vi "pessimize_adjust_bias.vi"(10 "X at maximum":dbl[](array[numeric]), 11 "Pessimize fun info":T1 {"Point selector"."Light number" min=0 max=5}) -> (1 "f(X)":dbl, 2 "Error vector":dbl[](array[numeric]), 3 "Pose bias":dbl[](array[numeric]) format="%#_3p")   [LabVIEW 2013]
uses:
  pessimize_objective_fun_info.ctl
  calibration/point_selector.ctl
  ui_override_opts.ctl
  <vilib>/Analysis/Matrix/Datatypes/RealMatrix.ctl
  <vilib>/Analysis/baseanly.llb/Real A x B.vi
  <vilib>/Analysis/NI_AALBase.lvlib
  <vilib>/Analysis/Matrix/NI_Matrix.lvlib
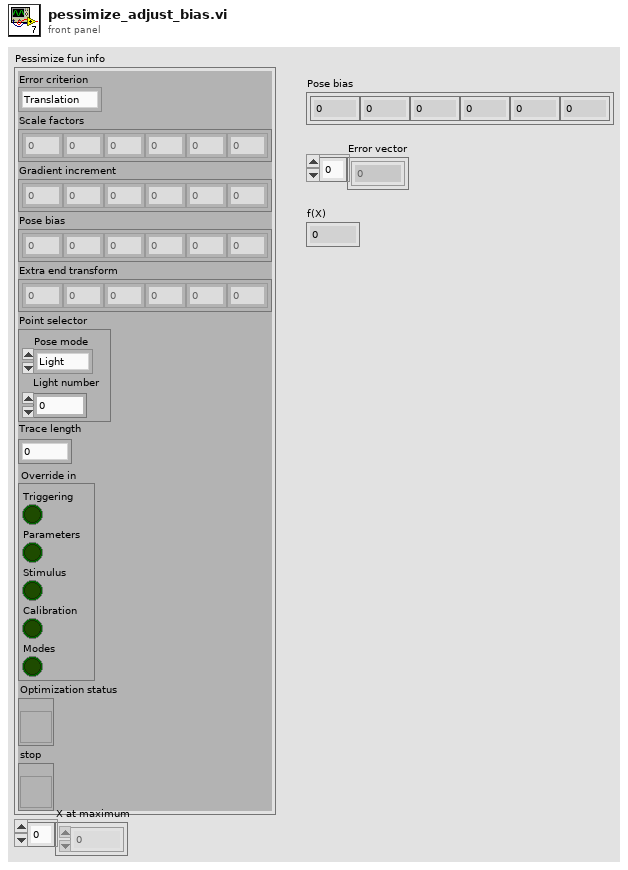
[diagram p1: front panel]
types:
  T1 = typedef "pessimize_objective_fun_info.ctl" = cluster{"Error criterion":enum16{"Translation", "Orientation", "Moment"}, "Scale factors":dbl[], "Gradient increment":dbl[], "Pose bias":dbl[], "Extra end transform":dbl[], "Point selector":T2, "Trace length":dbl, "Override in":T3, "Optimization status":refnum<vi>, "stop":refnum<vi>}
  T2 = typedef "point_selector.ctl" = cluster{"Pose mode":enum16{"Light", "Handle", "Output"}, "Light number":i32}
  T3 = typedef "ui_override_opts.ctl" = cluster{"Triggering":bool, "Parameters":bool, "Stimulus":bool, "Calibration":bool, "Modes":bool}
  T4 = typedef "NI_Matrix.lvlib/RealMatrix.ctl" = dbl[][]
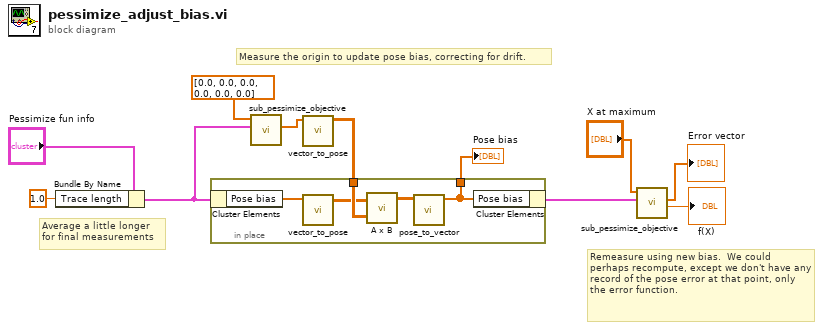
[diagram p0: block diagram]
diagram:
  # "Remeasure using new bias.  We could perhaps recompute, except we don't have any record of the pose error at that point, only the error function."
  # "Average a little longer \nfor final measurements"
  # "Measure the origin to update pose bias, correcting for drift."
  n1 = Bundle By Name(cluster="Pessimize fun info", "Trace length"=1.0) -> (w11:T1)
  n2 = call "sub_pessimize_objective.vi"("Pessimize fun info"=w11, "X"=dbl[] [0.0, 0.0, 0.0, 0.0, 0.0, 0.0]) -> ("Error vector"=w5:dbl[])  [unwired: 6 in, 3 out]
  n3 = call "vector_to_pose.vi"("Pose vector"=w5) -> ("Pose"=w6:T4)  [unwired: 10 in]
  n4 = in-place {
    in-place-border: w6 -> [w15]
    in-place-border: [w12] -> w7
    n5 = in-place-cluster #1(w11) -> ("Pose bias"=w16:dbl[])
    n6 = call "vector_to_pose.vi"("Pose vector"=w16) -> ("Pose"=w14:T4)  [unwired: 10 in]
    n7 = call-poly <vilib>:"A x B.vi"("B"=w15, "A"=w14) -> ("A x B"=w13:T4)  [unwired: 1 out]
    n8 = call "pose_to_vector.vi"("Pose"=w13) -> ("Pose vector"=w12:dbl[])  [unwired: 10 in]
    n9 = in-place-cluster #1("Pose bias"=w12) -> (w4:T1)
  }
  "Pose bias" <- w7
  n10 = call "sub_pessimize_objective.vi"("Pessimize fun info"=w4, "X"="X at maximum") -> ("f(X)"=→"f(X)":dbl, "Error vector"=→"Error vector":dbl[])  [unwired: 6 in, 2 out]
